vi "find_patches_lvalt.vi"() -> ()   [LabVIEW 2017, in "gVision.lvlib"]
uses:
  gVision.lvlib
  <vilib>/vision/NI_Vision_Development_Module.lvlib
  <vilib>/vision/Image Controls.llb/IMAQ Image.ctl
  find_patches parameters.ctl
  Vision.lvlib
panel:
  in  "Numeric":i32=2
  out "Lookup Table":i32[](array[numeric]) min=0 max=255
  out "Threshold Data out":T1(array[cluster]) {"Replace Value" format="%.2f"; "Upper value" format="%.2f"; "Lower value" format="%.2f"}
  out "Image 2":T2(plugin-control)
  in  "File Path":path
  in  "Field of View":cluster{"fieldOfViewX":sgl, "fieldOfViewY":sgl}
  out "Patches":T3(array[cluster])
  in  "Shrink Factor":i32=1
  in  "find_patches parameters":T4
  in  "Log File Directory":string
  in  "debug":bool
  in  "Image":T2
  out "error out":errorcluster
  in  "error in":errorcluster
  # "Image must be an 8-bin greyscale image"
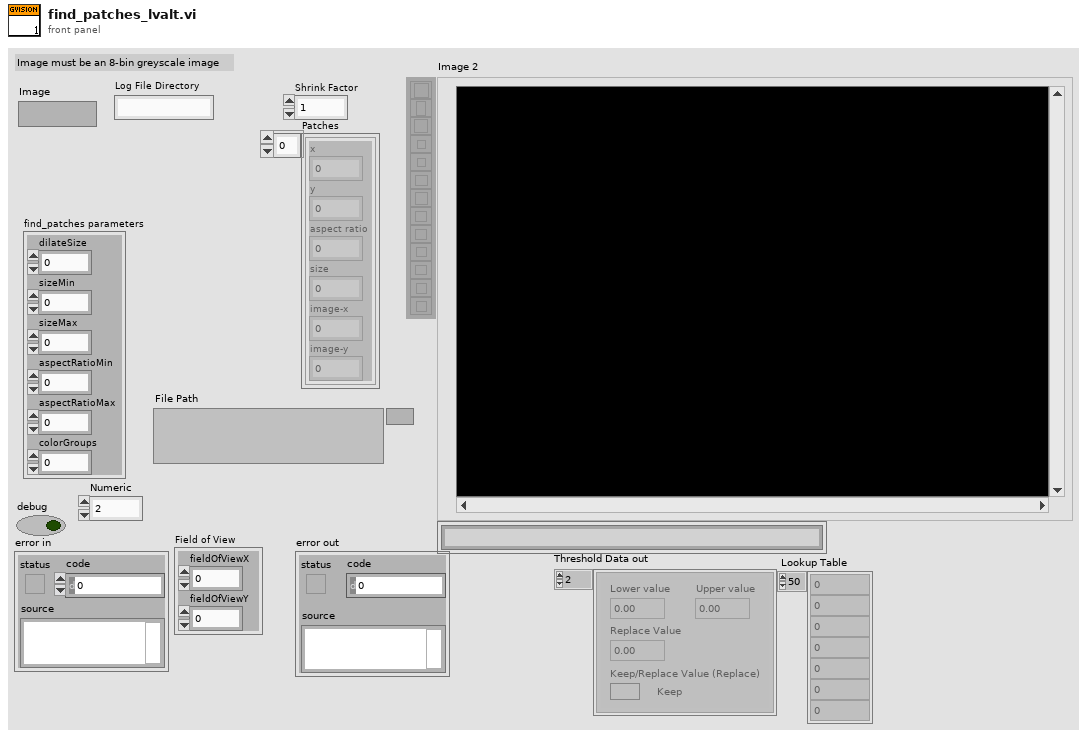
[diagram p1: front panel]
types:
  T1 = cluster{"Lower value":sgl, "Upper value":sgl, "Replace Value":sgl, "Keep/Replace Value (Replace)":bool}[]
  T2 = typedef "IMAQ Image.ctl" = refnum<image>
  T3 = cluster{"x":dbl, "y":dbl, "aspect ratio":dbl, "size":dbl, "image-x":dbl, "image-y":dbl}[]
  T4 = typedef "Vision.lvlib/find_patches parameters.ctl" = cluster{"dilateSize":i32, "sizeMin":sgl, "sizeMax":sgl, "aspectRatioMin":sgl, "aspectRatioMax":sgl, "colorGroups":i32}
  T5 = cluster{"Lower value":sgl, "Upper value":sgl, "Replace Value":sgl, "Keep/Replace Value (Replace)":bool}
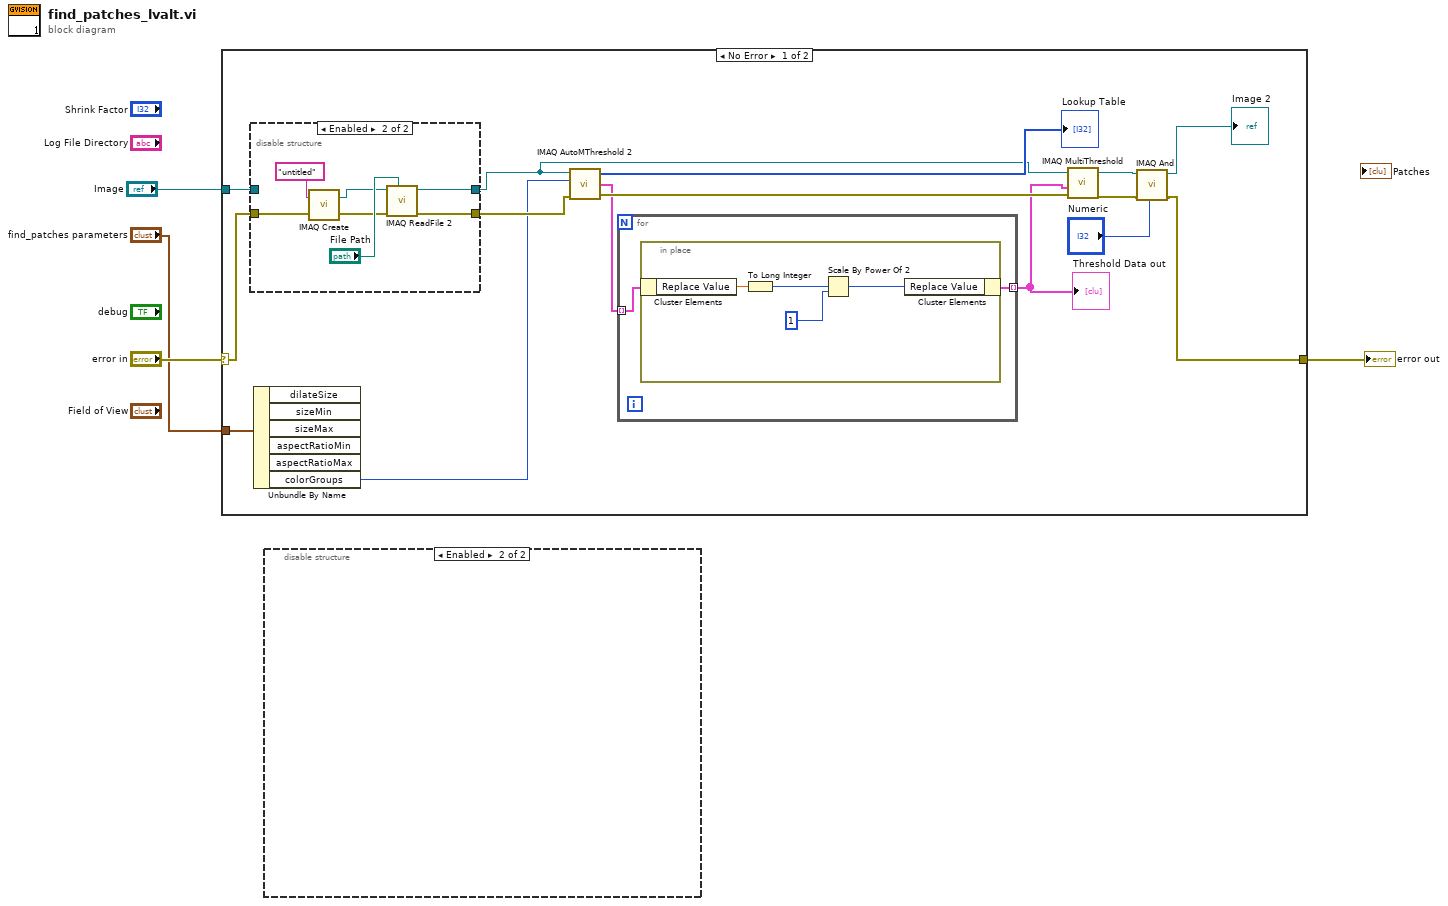
[diagram p0: block diagram]
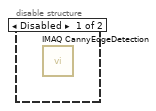
[diagram p4: hidden frame]
diagram:
  n1 = case shown="No Error" "error in" {
    selector: "error in" -> [w18 w35]
    tunnel: [w9 w35] -> w3
    tunnel: "Image" -> [w19 _]
    tunnel: "find_patches parameters" -> [w16 _]
    frame No Error {
      n2 = disable-structure shown="Enabled" {
        disable-tunnel: w19 -> [w27 _]
        disable-tunnel: [w27 w34] -> w13
        disable-tunnel: w18 -> [w26 w31]
        disable-tunnel: [w26 w32] -> w17
        frame Disabled {
        }
        frame Enabled {
          n3 = call "IMAQ Create"("Image Name"="untitled", "error in (no error)"=w31) -> ("New Image"=w29:T2, "error out"=w30:errorcluster)  [unwired: 3 in]
          n4 = call "IMAQ ReadFile 2"("File Path"="File Path", "error in (no error)"=w30, "Image"=w29) -> ("error out"=w32:errorcluster, "Image Out"=w34:T2)  [unwired: 4 in, 3 out]
        }
      }
      n5 = Unbundle By Name(w16) -> ("colorGroups"=w15:i32)  [unwired: 5 out]
      n6 = call "IMAQ AutoMThreshold 2"("error in (no error)"=w17, "Number of Classes"=w15, "Image"=w13) -> ("error out"=w12:errorcluster, "Threshold Data out"=w6:T1, "Lookup Table"=→"Lookup Table":i32[])  [unwired: 1 in]
      n7 = for {
        tunnel: w6 -> [w21] mode=indexing
        tunnel: [w20] -> w5 mode=indexing
        n8 = in-place {
          n9 = in-place-cluster #1(w21) -> ("Replace Value"=w25:sgl)
          n10 = To Long Integer(number=w25) -> (32bit integer=w23:i32)
          n11 = Scale By Power Of 2(n=w23, x=i16 1 ("n")) -> (x*2^n=w24:i16)
          n12 = in-place-cluster #1("Replace Value"=w24) -> (w20:T5)
        }
      }
      "Threshold Data out" <- w5
      n13 = call "IMAQ MultiThreshold"("error in (no error)"=w12, "Threshold Data"=w5, "Image Src"=w13) -> ("error out"=w10:errorcluster, "Image Dst Out"=w11:T2)  [unwired: 2 in]
      n14 = call "IMAQ And"("Constant"="Numeric", "error in (no error)"=w10, "Image Src A"=w11) -> ("error out"=w9:errorcluster, "Image Dst Out"=→"Image 2":T2)  [unwired: 7 in]
    }
    frame Error {
    }
  }
  "error out" <- w3
  n15 = disable-structure shown="Enabled" {
    frame Disabled {
      n16 = call "IMAQ CannyEdgeDetection"() -> ()  [unwired: 8 in, 2 out]
    }
    frame Enabled {
    }
  }
